vi "V1.0_UI.vi"() -> ()   [LabVIEW 2018]
uses:
  lib/Olympus IX BX Series/Olympus IX BX Series.lvlib
  <vilib>/MakerHub/LINX/LMH-LINX.lvlib
  lib/ARDUINO/VIs/Arduino.lvlib
  lib/SOLA/LabVIEW 2015 Library (32bit)/LumencorDLL32/LumencorDLL32.lvlib
  lib/TANGO Stage/TangoOWN.lvlib
  <userlib>/Tango_DLL/Tango_DLL.lvlib
  lib/ANDOR/Andor SDK/AndorSDK.lvlib
  lib/ANDOR/OwnVIs/AndorOWN.lvlib
  <vilib>/vision/NI_Vision_Development_Module.lvlib
  <vilib>/MakerHub/LINX/Public/Utilities/Open Serial.vi
  <vilib>/Utility/inputDevices.llb/closeKeyboard.vi
  <vilib>/Utility/inputDevices.llb/keyboardAcquire.vi
panel:
  in  "Filter":u16(ring) items=["UV ", "CFP", "GFP", "YFP", "RFP", "BF (empty)"]
  in  "Exposure":sgl=50.0 format="%#_g ms"
  out "exposure out":sgl
  out "accumulate out":sgl
  out "kinetic out":sgl
  out "Camera Temperature":sgl format="%.2f °C"
  in  "Single/\nMultiring?":bool
  in  "Image Name":string="TestIMG"
  out "Acq. Error Array":cluster{i32, string}[](array[cluster])
  in  "Live Mode":bool
  in  "Single Image":bool
  in  "Calibrate at Startup":bool
  out "keys pressed":T1(array[ring])
  out "Position List":i32[](listbox)
  in  "Down":bool
  in  "Left":bool
  in  "Up":bool
  in  "Right":bool
  in  "Clear Last Pos":bool
  in  "Save Pos":bool
  out "Boolean":bool
  in  "TANGO COM Port":refnum<visa-resource-name>="COM4"
  in  "SOLA COM Port":u32=5 max=10 step=1
  in  "Valve Port (Arduino)":refnum<visa-resource-name>="COM7"
  in  "IX 81 Port (IX2 UCB)":refnum<visa-resource-name>="IX2-UCB"
  out "Tango Connection\n Error":i32
  out "Y Limits":dbl[](array[numeric]) caption="Y Limits [µm]" format="%#_12f"
  out "X Limits":dbl[](array[numeric]) caption="X Limits [µm]" format="%#_10f"
  in  "Step Width [µm]":dbl=100.0 min=0.0 format="%#_6f"
  out "Position":dbl[](array[numeric]) caption="Position [µm]" format="%#_12f"
  out "Current z-Position":dbl
  in  "Direction (1: Down)":enum16{"Up", "Down", "Abs"}(ring)=enum."Abs"
  in  "Step (0.0 um)":dbl format="%.1f"
  out "Upper Limit":dbl
  out "Lower Limit":dbl
  in  "Light Source":u16(ring) items=["BF - Lamp", "SOLA"]
  in  "Intensity [%]":dbl(slide) scale=0.0..100.0 scale format="%.1f"
  in  "Prism Position (1: Bi)":enum16{"Bi", "Side"}(ring)=enum."Side"
  in  "Objective":enum16{"x 4", "x 10", "x 20", "x 40", "x 100"}(ring)=enum."x 10"
  in  "Shutter":bool
  in  "Enable Lamp":bool
  in  "Lamp Type (0: Transmitted)":enum16{"Transmitted", "Reflected"}(ring)
  out "Info":string caption="String"
  out "Image":T2(plugin-control)
  out "error out":errorcluster
  in  "Flush\nReagent":u16
  in  "Flush":bool
  in  "Pump Cycles":dbl=20.0
  in  "Frequency":dbl=50.0 format="%#_3f"
  in  "Pump On":bool
  in  "Feed On":bool
  in  "Feed Cycles":i32=20
  in  "Feed\nReagent":u16=2
  in  "Ring":u16
  in  "All Rings":bool
  in  "stop":bool
  # "Stage"
  # "X"
  # "Y"
  # "min"
  # "min"
  # "max"
  # "max"
  # "S"
  # "M"
  # "Initialization"
  # "Microscope"
  # "Valve Functions"
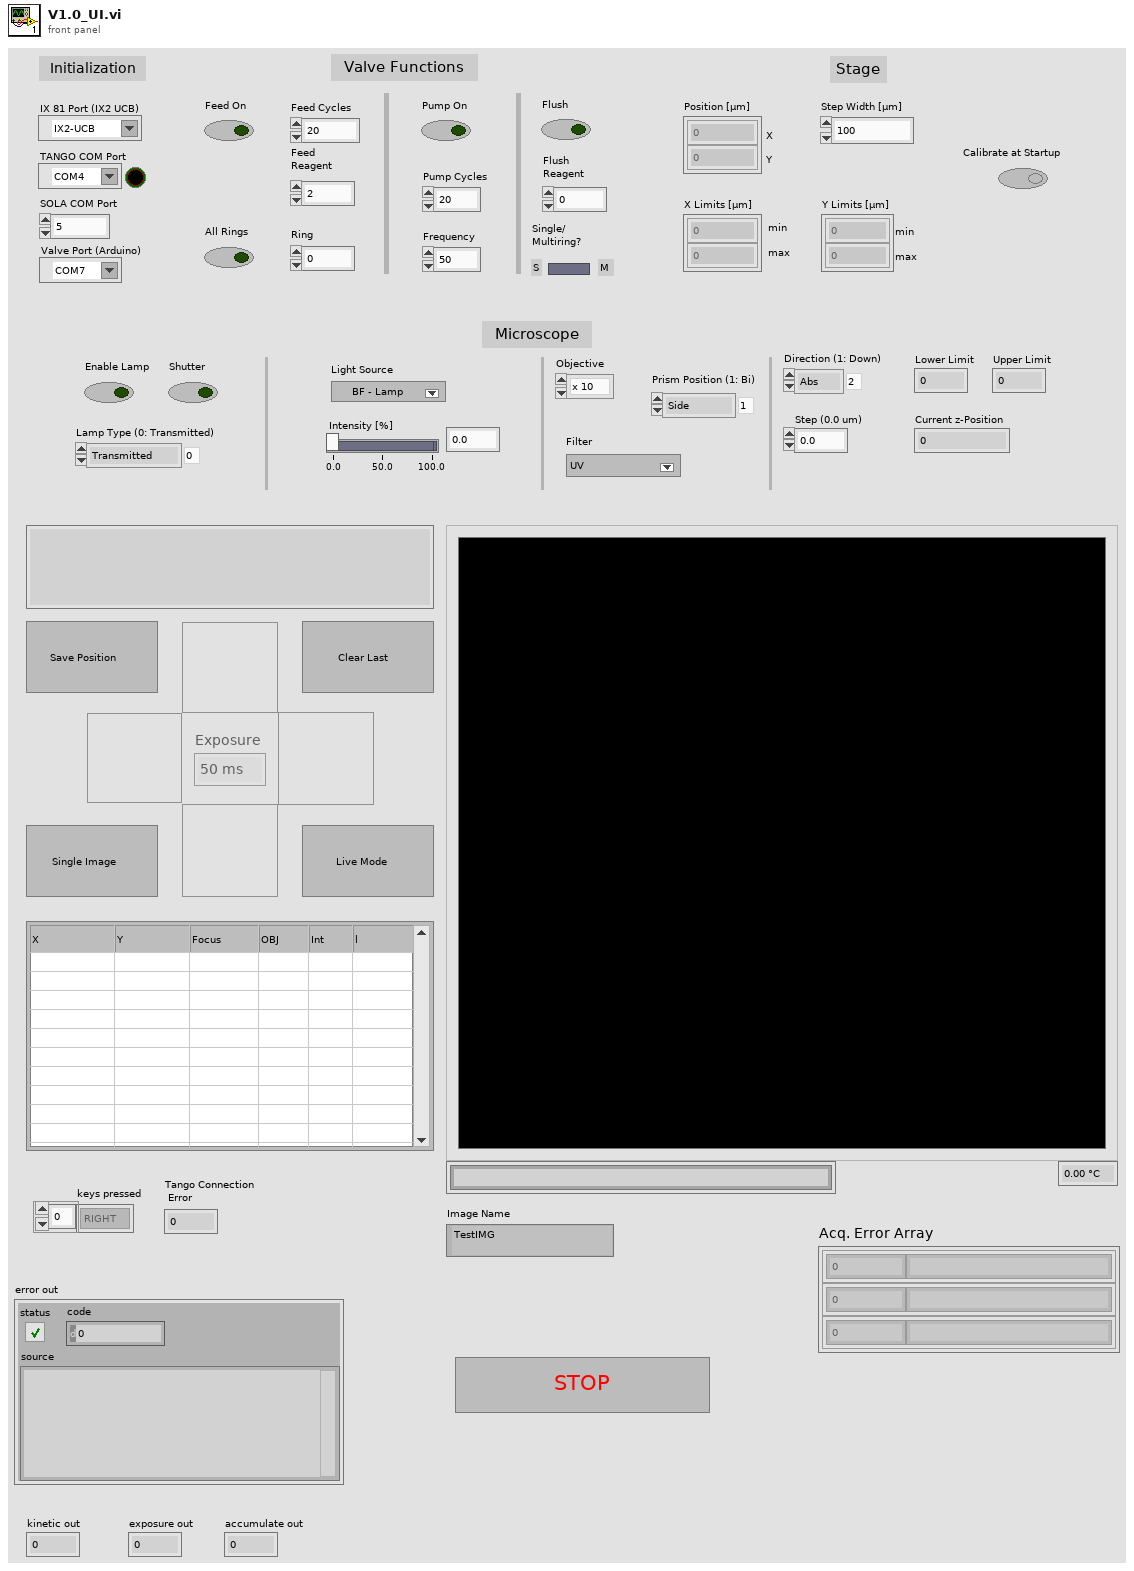
[diagram p1: front panel]
types:
  T1 = enum16{"0", "1", "2", "3", "4", "5", "6", "7", "8", "9", "A", "B", "C", "D", "E", "F", "G", "H", "I", "J", "K", "L", "M", "N", "O", "P", "Q", "R", "S", "T", "U", "V", "W", "X", "Y", "Z", "F1", "F2", "F3", "F4", "F5", "F6", "F7", "F8", "F9", "F10", "F11", "F12", "F13", "F14", "F15", "ADD", "BACK", "BACKSLASH", "CAPITAL", "COMMA", "DECIMAL", "DELETE", "DIVIDE", "DOWN", "END", "EQUALS", "ESCAPE", "GRAVE (`)", "HOME", "INSERT", "LBRACKET", "LCONTROL", "LEFT", "L ALT", "LSHIFT", "LWIN", "MINUS", "MULTIPLY", "NEXT", "NUMLOCK", "NUMPAD_0", "NUMPAD_1", "NUMPAD_2", "NUMPAD_3", "NUMPAD_4", "NUMPAD_5", "NUMPAD_6", "NUMPAD_7", "NUMPAD_8", "NUMPAD_9", "PAUSE", "PERIOD", "PRIOR (PG UP)", "RBRACKET", "RCONTROL", "RETURN", "RIGHT", "R ALT", "RSHIFT", "RWIN", "SCROLL", "SEMICOLON", "SLASH", "SPACE", "SUBTRACT", "TAB", "UP", "ENTER (num pad)", "' (quote)"}[]
  T2 = typedef "IMAQ Image.ctl" = refnum<image>
  T3 = enum32{"UV", "CFP", "GFP", "YFP", "RFP", "BF (empty)"}
  T4 = typedef "LMH-LINX.lvlib/LINX Ref.ctl" = cluster{"IO":T5, "Interface":T6, "LINX Device Config":T7}
  T5 = typedef "LMH-LINX.lvlib/Platform.ctl" = enum16{"Remote", "Local"}
  T6 = typedef "LMH-LINX.lvlib/Interface.ctl" = enum16{"Serial", "TCP"}
  T7 = typedef "LMH-LINX.lvlib/Device.lvlib/LINX Device Config.ctl" = cluster{"Interface":T6, "COM Port":refnum<visa-resource-name>, "TCP Configuration":T8, "Device Family":u8, "Device ID":u8, "Device Name":string, "TCP Ref":refnum<k5>, "Channels":T9}
  T8 = typedef "LMH-LINX.lvlib/Device.lvlib/TCP Config.ctl" = cluster{"IP Address":string, "Port":u16}
  T9 = typedef "LMH-LINX.lvlib/Channels.ctl" = cluster{"DI":u8[], "DO":u8[], "AI":u8[], "AO":u8[], "PWM":u8[], "QE":u8[], "UART":u8[], "I2C 2":u8[], "SPI":u8[], "CAN":u8[], "Servo":u8[], "AI Ref (V)":dbl, "AI Resolution (Bits)":u8, "AO Ref (V)":dbl, "AO Resolution (Bits)":u8}
  T10 = cluster{"X":dbl, "Y\nY":dbl, "Focus":dbl, "Objective":string, "filter":string, "Intensity":dbl}[]
  T11 = cluster{"pdX out":dbl, "pdY out":dbl, dbl, string, string, "Value":dbl}
  T12 = cluster{"pdX out":dbl, "pdY out":dbl, "Focus":dbl, "Objective":string, "filter":string, "Value":dbl}[]
  T13 = enum8{"Enabled", "Disabled", "Disabled and Grayed Out"}
  T14 = typedef "Image Type" = u32
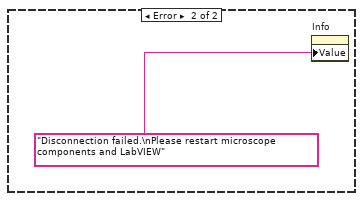
[diagram p2: hidden frame]
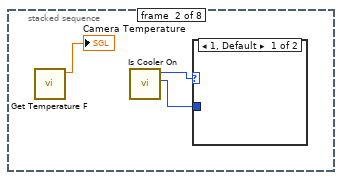
[diagram p3: hidden frame]
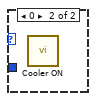
[diagram p4: hidden frame]
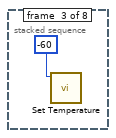
[diagram p5: hidden frame]
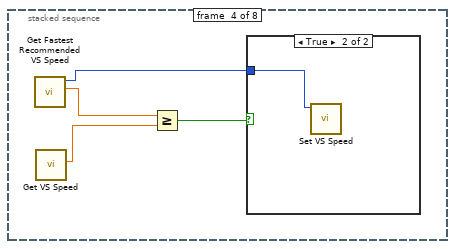
[diagram p6: hidden frame]
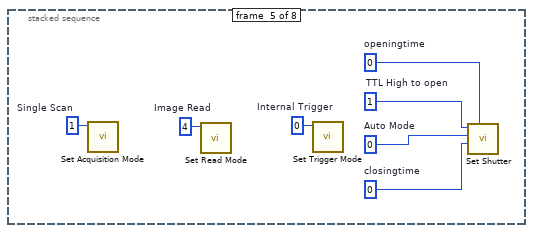
[diagram p8: hidden frame]
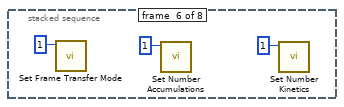
[diagram p9: hidden frame]
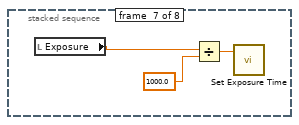
[diagram p10: hidden frame]
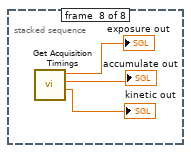
[diagram p11: hidden frame]
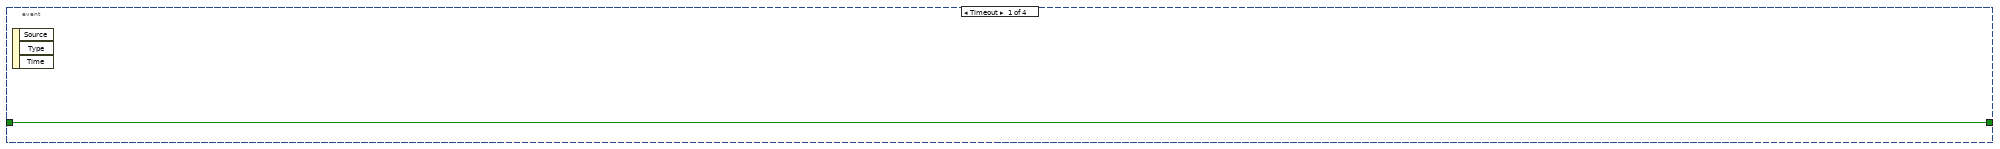
[diagram p12: hidden frame]
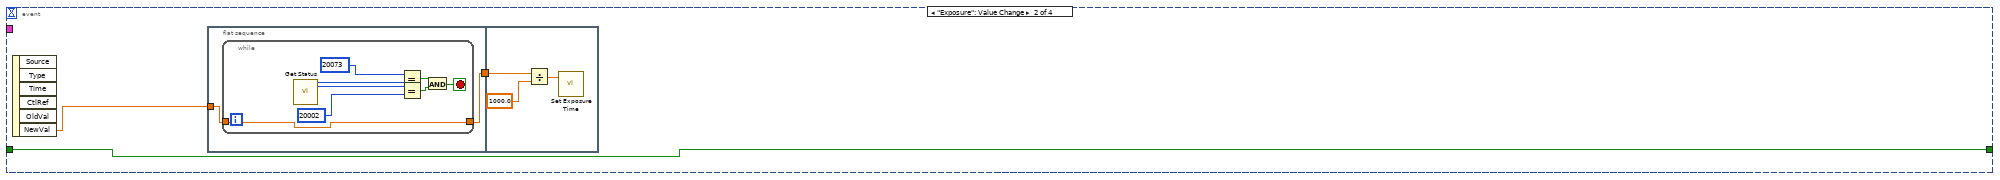
[diagram p13: hidden frame]
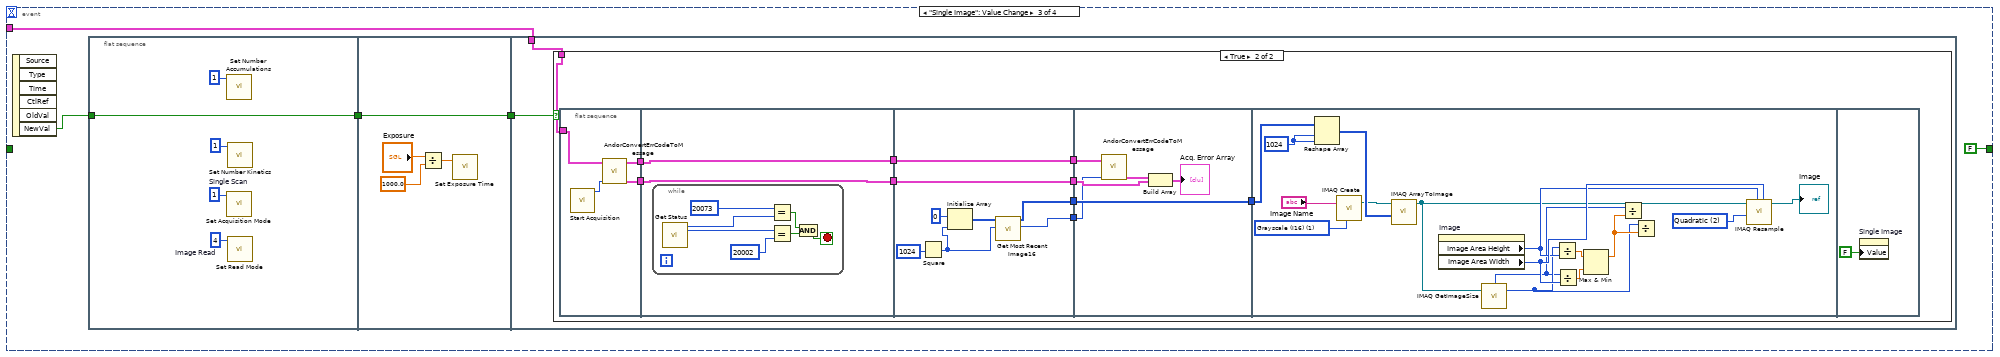
[diagram p14: hidden frame]
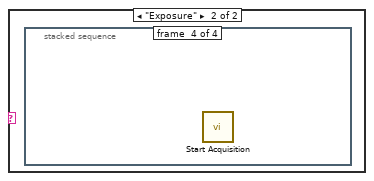
[diagram p17: hidden frame]
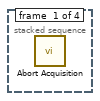
[diagram p18: hidden frame]
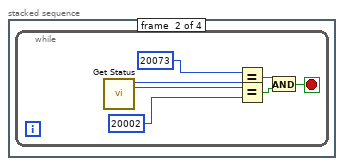
[diagram p19: hidden frame]
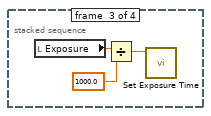
[diagram p20: hidden frame]
diagram:
  n1 = flat-sequence {
    tunnel: [w46] -> w22
    tunnel: [w47] -> w21
    tunnel: [w51] -> w20
    tunnel: [w43] -> w19
    tunnel: [w41] -> w18
    tunnel: w22 -> [w74]
    tunnel: [w74] -> w17
    tunnel: w21 -> [w73]
    tunnel: [w73] -> w15
    tunnel: w20 -> [w72]
    tunnel: [w72] -> w12
    tunnel: w19 -> [w71]
    tunnel: [w71] -> w10
    tunnel: w18 -> [w70]
    tunnel: [w70] -> w8
    tunnel: w17 -> [w81]
    tunnel: [w81] -> w16
    tunnel: w15 -> [w80]
    tunnel: [w80] -> w14
    tunnel: [w75] -> w13
    tunnel: w12 -> [w79]
    tunnel: [w79] -> w11
    tunnel: w10 -> [w78]
    tunnel: [w78] -> w9
    tunnel: w8 -> [w77]
    tunnel: w16 -> [w90]
    tunnel: [w104] -> w34
    tunnel: w14 -> [w172]
    tunnel: [w172] -> w32
    tunnel: w13 -> [w89]
    tunnel: [w96] -> w30
    tunnel: w11 -> [w171]
    tunnel: [w171] -> w28
    tunnel: w9 -> [w94]
    tunnel: [w94] -> w26
    tunnel: w34 -> [w195]
    tunnel: [w195] -> w33
    tunnel: w32 -> [w194]
    tunnel: [w194] -> w31
    tunnel: w30 -> [w189]
    tunnel: [w191] -> w29
    tunnel: w28 -> [w193]
    tunnel: [w193] -> w27
    tunnel: w26 -> [w192]
    tunnel: [w192] -> w25
    tunnel: [w187] -> w24
    tunnel: w33 -> [w209]
    tunnel: w31 -> [w207]
    tunnel: w29 -> [w208]
    tunnel: [w206] -> w39
    tunnel: [w205] -> w38
    tunnel: [w204] -> w37
    tunnel: w27 -> [w203]
    tunnel: [w202] -> w36
    tunnel: w25 -> [w200]
    tunnel: [w201] -> w35
    tunnel: w24 -> [w199]
    tunnel: [w198] -> w23
    tunnel: w39 -> [w785]
    tunnel: w38 -> [w779]
    tunnel: w37 -> [w771]
    tunnel: [w770] -> w4
    tunnel: w36 -> [w772]
    tunnel: w35 -> [w773]
    tunnel: w23 -> [w774]
    frame #0 {
      "Info" <- "Connecting..." ("Info")
    }
    frame #1 {
      w62 = 2  # Device Number (1: -Condensor      - Objective      - Lamp      - Shutter 2: - Z-Motion    - Autofocus)
      w61 = 1  # Device Number (1: -Condensor      - Objective      - Lamp      - Shutter 2: - Z-Motion    - Autofocus)
      n2 = call "Initialize.vi"("VISA Resource Name"="IX 81 Port (IX2 UCB)") -> ("VISA Resource Name Out"=w68:refnum<visa-resource-name>, "error out"=w67:errorcluster)  [unwired: 13 in]
      n3 = call "Login Device.vi"("error in (no error)"=w67, "Device Number (1)"=w61, "VISA Resource Name"=w68) -> ("error out"=w65:errorcluster, "VISA Resource Name Out"=w66:refnum<visa-resource-name>)  [unwired: 7 in]
      n4 = call "Login Device.vi"("error in (no error)"=w65, "Device Number (1)"=w62, "VISA Resource Name"=w66) -> ("error out"=w63:errorcluster, "VISA Resource Name Out"=w46:refnum<visa-resource-name>)  [unwired: 7 in]
      n5 = call-poly <vilib>:"Open.vi"("Error In"=w63, "Serial Port"="Valve Port (Arduino)") -> ("Error Out"=w60:errorcluster, "LINX Resource"=w47:T4)  [unwired: 7 in, 1 out]
      n6 = Decrement(x="SOLA COM Port") -> (x-1=w50:u32)
      n7 = call "lm Init.vi"("error in (no error)"=w60, "LETypeStr"="SOLA", "ComPort"=w50) -> ("error out"=w57:errorcluster, "function return"=w51:u32)  [unwired: 6 in, 1 out]
      n8 = call "lm Color Level.vi"("error in (no error)"=w57, "str_Level"="0", "str_Color"="WHITE") -> ("error out"=w53:errorcluster, "str_Color out"=w54:string)  [unwired: 6 in, 1 out]
      n9 = call "lm Color Enable.vi"("error in (no error)"=w53, "str_State"="OFF", "str_Color"=w54) -> ("error out"=w48:errorcluster)  [unwired: 6 in, 2 out]
      n10 = property on="Boolean" class="Bool (strict)"("Colors [4]"=cluster{u32, u32}[] [{16711680, 0}, {65280, 0}, {6710886, 0}, {6710886, 0}]) -> ()  [unwired: 2 in, 2 out]
      n11 = call "TangoConnectSub.vi"("error in (no error)"=w48, "VISA Refnum in"="TANGO COM Port") -> ("error out"=w41:errorcluster, "function return"=w45:i32, "plLSID out"=w43:i32)  [unwired: 7 in]
      "Tango Connection\n Error" <- w45
      n12 = Equal To 0?(x=w45) -> (x = 0?=→"Boolean":bool)
    }
    frame #2 {
    }
    frame #3 {
      n13 = property on="Info" class="Str"(error in=w77, "Value"="Connection to all devices successful." ("Info")) -> (error out=w75:errorcluster)  [unwired: 1 in, 1 out]
    }
    frame #4 {
      n14 = call "Set Active Objective.vi"("error in (no error)"=w89, "Objective Number (1)"=1, "Device Number (1)"=1, "VISA Resource Name"=w90) -> ("error out"=w92:errorcluster, "VISA Resource Name Out"=w91:refnum<visa-resource-name>)  [unwired: 6 in]
      n15 = case shown="True" "Calibrate at Startup" {
        tunnel: w94 -> [_ w180]
        tunnel: [w173 w179] -> w93
        tunnel: w92 -> [w173 w178]
        tunnel: [dbl[] [0.0, 80674.8] ("Y Limits") w177] -> w86
        tunnel: [dbl[] [0.0, 120822.0] ("X Limits") w176] -> w85
        frame False {
        }
        frame True {
          n16 = call "TangoCalibrate.vi"("error in (no error)"=w178, "plLSID in"=w180) -> ("error out"=w179:errorcluster, "X Limits"=w176:dbl[], "Y Limits"=w177:dbl[])  [unwired: 7 in]
        }
      }
      "X Limits" <- w85
      "Y Limits" <- w86
      n17 = call "OlympusQuery.vi"("error in (no error)"=w93, "Device Number\n(1: -Condensor\n     - Objective\n     - Lamp\n     - Shutter\n2: - Z-Motion\n   - Autofocus)"=1 ("Device Number\n(1: -Condensor\n     - Objective\n     - Lamp\n     - Shutter\n2: - Z-Motion\n   - Autofocus)"), "String"="SW OFF", "VISA Resource Name In"=w91) -> ("error out"=w101:errorcluster, "VISA Resource Name Out"=w102:refnum<visa-resource-name>)  [unwired: 5 in, 1 out]
      n18 = call "OlympusQuery.vi"("error in (no error)"=w101, "String"="LMPSW?", "VISA Resource Name In"=w102) -> ("error out"=w170:errorcluster, "Result"=w137:string, "VISA Resource Name Out"=w165:refnum<visa-resource-name>)  [unwired: 6 in]
      n19 = Equal?(x=w137, y="ON") -> (x = y?=w136:bool)
      n20 = property on="Enable Lamp" class="Bool (strict)"(error in=w170, "Value"=w136) -> (error out=w168:errorcluster)  [unwired: 1 in, 1 out]
      n21 = call "OlympusQuery.vi"("error in (no error)"=w168, "String"="LMP?", "VISA Resource Name In"=w165) -> ("error out"=w167:errorcluster, "Result"=w106:string, "VISA Resource Name Out"=w162:refnum<visa-resource-name>)  [unwired: 6 in]
      n22 = Decimal String To Number(string=w106, default (0L)=0.0 ("default (0 I32)")) -> (number=w108:dbl)  [unwired: 1 in, 1 out]
      n23 = Divide(x=w108, y=1.2 ("x")) -> (x/y=w134:dbl)
      n24 = property on="Intensity [%]" class="Slide (strict)"(error in=w167, "Value"=w134) -> (error out=w164:errorcluster)  [unwired: 1 in, 1 out]
      n25 = call "OlympusQuery.vi"("error in (no error)"=w164, "String"="SHUT1?", "VISA Resource Name In"=w162) -> ("error out"=w163:errorcluster, "Result"=w133:string, "VISA Resource Name Out"=w158:refnum<visa-resource-name>)  [unwired: 6 in]
      n26 = Equal?(x=w133, y="OUT") -> (x = y?=w131:bool)
      n27 = property on="Shutter" class="Bool (strict)"(error in=w163, "Value"=w131) -> (error out=w160:errorcluster)  [unwired: 1 in, 1 out]
      n28 = call "OlympusQuery.vi"("error in (no error)"=w160, "String"="LMPSEL?", "VISA Resource Name In"=w158) -> ("error out"=w159:errorcluster, "Result"=w130:string, "VISA Resource Name Out"=w155:refnum<visa-resource-name>)  [unwired: 6 in]
      n29 = Equal?(x=w130, y="DIA") -> (x = y?=w128:bool)
      n30 = Not(x=w128) -> (.not. x?=w127:bool)
      n31 = Boolean To (0,1)(Boolean=w127) -> (0, 1=w126:i16)
      n32 = property on="Lamp Type\n (0: Transmitted)" class="Enum (strict)"(error in=w159, "Value"=w126) -> (error out=w156:errorcluster)  [unwired: 1 in, 1 out]
      n33 = call "OlympusQuery.vi"("error in (no error)"=w156, "String"="MU?", "VISA Resource Name In"=w155) -> ("error out"=w82:errorcluster, "Result"=w125:string, "VISA Resource Name Out"=w98:refnum<visa-resource-name>)  [unwired: 6 in]
      n34 = Decimal String To Number(string=w125) -> (number=w124:i32)  [unwired: 2 in, 1 out]
      n35 = Decrement(x=w124) -> (x-1=w83:i32)
      n36 = local write "Filter"(w83) -> ()
      n37 = case shown="0, Default" w83 {
        tunnel: w82 -> [w182 w185]
        tunnel: [w181 w184] -> w97
        frame 0, Default {
          w183 = u16 1 items=["BF - Lamp", "SOLA"] ("Light Source")
          n38 = property on="Light Source" class="Ring (strict)"(error in=w182, "Value"=w183) -> (error out=w181:errorcluster)  [unwired: 1 in, 1 out]
        }
        frame 5 {
          w186 = u16 0 items=["BF - Lamp", "SOLA"] ("Light Source")
          n39 = property on="Light Source" class="Ring (strict)"(error in=w185, "Value"=w186) -> (error out=w184:errorcluster)  [unwired: 1 in, 1 out]
        }
      }
      n40 = call "OlympusQuery.vi"("error in (no error)"=w97, "String"="OB?", "VISA Resource Name In"=w98) -> ("error out"=w153:errorcluster, "Result"=w123:string, "VISA Resource Name Out"=w148:refnum<visa-resource-name>)  [unwired: 6 in]
      n41 = Decimal String To Number(string=w123) -> (number=w122:i32)  [unwired: 2 in, 1 out]
      n42 = Decrement(x=w122) -> (x-1=w99:i32)
      n43 = property on="Objective" class="Enum (strict)"(error in=w153, "Value"=w99) -> (error out=w151:errorcluster)  [unwired: 1 in, 1 out]
      n44 = call "OlympusQuery.vi"("error in (no error)"=w151, "String"="PRISM?", "VISA Resource Name In"=w148) -> ("error out"=w150:errorcluster, "Result"=w121:string, "VISA Resource Name Out"=w146:refnum<visa-resource-name>)  [unwired: 6 in]
      n45 = Decimal String To Number(string=w121) -> (number=w120:i32)  [unwired: 2 in, 1 out]
      n46 = Decrement(x=w120) -> (x-1=w119:i32)
      n47 = property on="Prism Position\n (1: Bi)" class="Enum (strict)"(error in=w150, "Value"=w119) -> (error out=w147:errorcluster)  [unwired: 1 in, 1 out]
      n48 = call "OlympusQuery.vi"("error in (no error)"=w147, "Device Number\n(1: -Condensor\n     - Objective\n     - Lamp\n     - Shutter\n2: - Z-Motion\n   - Autofocus)"=2 ("Device Number\n(1: -Condensor\n     - Objective\n     - Lamp\n     - Shutter\n2: - Z-Motion\n   - Autofocus)"), "String"="FARLMT 10", "VISA Resource Name In"=w146) -> ("error out"=w143:errorcluster, "VISA Resource Name Out"=w144:refnum<visa-resource-name>)  [unwired: 5 in, 1 out]
      n49 = call "OlympusQuery.vi"("error in (no error)"=w143, "Device Number\n(1: -Condensor\n     - Objective\n     - Lamp\n     - Shutter\n2: - Z-Motion\n   - Autofocus)"=2 ("Device Number\n(1: -Condensor\n     - Objective\n     - Lamp\n     - Shutter\n2: - Z-Motion\n   - Autofocus)"), "String"="NEARLMT 3000000", "VISA Resource Name In"=w144) -> ("error out"=w140:errorcluster, "VISA Resource Name Out"=w141:refnum<visa-resource-name>)  [unwired: 5 in, 1 out]
      n50 = call "OlympusQuery.vi"("error in (no error)"=w140, "Device Number\n(1: -Condensor\n     - Objective\n     - Lamp\n     - Shutter\n2: - Z-Motion\n   - Autofocus)"=2 ("Device Number\n(1: -Condensor\n     - Objective\n     - Lamp\n     - Shutter\n2: - Z-Motion\n   - Autofocus)"), "String"="POS?", "VISA Resource Name In"=w141) -> ("error out"=w112:errorcluster, "Result"=w113:string, "VISA Resource Name Out"=w111:refnum<visa-resource-name>)  [unwired: 5 in]
      n51 = Decimal String To Number(string=w113, default (0L)=0.0 ("default (0 I32)")) -> (number=→"Current z-Position":dbl)  [unwired: 1 in, 1 out]
      n52 = call "Configure Jog.vi"("VISA Resource Name"=w111, "Device Number (1)"=2, "Enabled (False)"=TRUE, "error in (no error)"=w112) -> ("VISA Resource Name Out"=w104:refnum<visa-resource-name>, "error out"=w96:errorcluster)  [unwired: 10 in]
      "Lower Limit" <- 3000000.0 ("default (0 I32)")
      "Upper Limit" <- 10.0 ("Upper Limit")
    }
    frame #5 {
      n53 = call <vilib>:"Intialize Keyboard.vi"("error in (no error)"=w189) -> ("error out"=w188:errorcluster, "device ID"=w187:refnum<k1>)  [unwired: 9 in]
      n54 = property on="Info" class="Str"(error in=w188, "Value"="Initialization Finished") -> (error out=w191:errorcluster)  [unwired: 1 in, 1 out]
    }
    frame #6 {
      w196 = T10 []  # Saved Positions
      w197 = ""  # Current Button
      n55 = while {
        shift-right: [w210] -> w204
        shift-left: w208 -> [w246]
        shift-right: [w243] -> w206
        shift-left: w207 -> [w244]
        shift-right: [w245] -> w205
        shift-left: w209 -> [w247]
        tunnel: w203 -> [w242]
        tunnel: [w241] -> w202
        shift-right: [w235] -> w201
        shift-left: w200 -> [w234]
        shift-right: [w232] -> w198
        shift-left: w199 -> [w231]
        shift-right: [w223] -> _
        shift-left: w197 -> [w230]
        shift-right: [w211] -> _
        shift-left: w196 -> [w213]
        stop <- w248 stop-if-true
        n56 = flat-sequence {
          tunnel: w247 -> [w257]
          tunnel: w246 -> [w256]
          tunnel: [w255] -> w240
          tunnel: [w254] -> w239
          tunnel: w244 -> [w253]
          tunnel: [w253] -> w238
          tunnel: w242 -> [w252]
          tunnel: [w252] -> w237
          tunnel: w234 -> [w251]
          tunnel: [w251] -> w236
          tunnel: [w250] -> w233
          tunnel: w231 -> [w250]
          tunnel: w240 -> [w429]
          tunnel: [w429] -> w229
          tunnel: w239 -> [w426]
          tunnel: w238 -> [w428]
          tunnel: w237 -> [w430]
          tunnel: [w430] -> w228
          tunnel: w236 -> [w420]
          tunnel: [w428] -> w227
          tunnel: w233 -> [w427]
          tunnel: [w425] -> w232
          tunnel: w230 -> [w423]
          tunnel: [w422] -> w226
          tunnel: [w421] -> w225
          tunnel: [w420] -> w224
          tunnel: w229 -> [w545]
          tunnel: [w545] -> w222
          tunnel: w228 -> [w544]
          tunnel: [w544] -> w220
          tunnel: [w540] -> w218
          tunnel: w227 -> [w543]
          tunnel: [w543] -> w216
          tunnel: w226 -> [w542]
          tunnel: w225 -> [w541]
          tunnel: w224 -> [w540]
          tunnel: [w539] -> w223
          tunnel: [w537] -> w214
          tunnel: w222 -> [w626]
          tunnel: [w621] -> w221
          tunnel: w220 -> [w630]
          tunnel: [w630] -> w219
          tunnel: w218 -> [w625]
          tunnel: [w625] -> w217
          tunnel: w216 -> [w629]
          tunnel: [w629] -> w215
          tunnel: w214 -> [w627]
          tunnel: w213 -> [w628]
          tunnel: [w623] -> w211
          tunnel: [w622] -> w212
          tunnel: w221 -> [w708]
          tunnel: w219 -> [w705]
          tunnel: w217 -> [w704]
          tunnel: w215 -> [w710]
          tunnel: w212 -> [w707]
          tunnel: [w705] -> w241
          tunnel: [w709] -> w243
          tunnel: [w706] -> w210
          tunnel: [w708] -> w245
          tunnel: [w704] -> w235
          frame #0 {
            w258 = 2  # Device Number (1: -Condensor      - Objective      - Lamp      - Shutter 2: - Z-Motion    - Autofocus)
            w259 = 1  # Device Number (1: -Condensor      - Objective      - Lamp      - Shutter 2: - Z-Motion    - Autofocus)
            n57 = event shown="[8] \"Step (0.0 um)\": Value Change" {
              selector: _ -> [_ _ _ _ _ _ _ _ _]
              dyn-events: _ -> [_ _ _ _ _ _ _ _ _]
              timeout: 1 -> [_ _ _ _ _ _ _ _ _]
              tunnel: w257 -> [w264 w309 w329 w357 w362 w371 w375 w383 w414]
              tunnel: w259 -> [_ _ _ _ w360 w372 _ _ _]
              tunnel: w258 -> [_ _ _ _ _ _ _ _ w413]
              tunnel: [w263 w310 w323 w356 w364 w367 w377 w382 w411] -> w254
              tunnel: [w262 w309 w324 w357 w365 w368 w378 w385 w412] -> w255
              tunnel: w256 -> [w261 w311 w327 w356 w361 w370 w376 w384 w415]
              event "Enable Lamp": Value Change {
                n58 = event-data() -> ()  [unwired: 1 in, 6 out]
                n59 = case shown="True" "Enable Lamp" {
                  selector: "Enable Lamp" -> [w268 w301]
                  tunnel: w264 -> [w271 w305]
                  tunnel: w261 -> [w267 w296]
                  tunnel: [w270 w304] -> w263
                  tunnel: [w269 w303] -> w262
                  frame True {
                    n60 = case shown="1" "Light Source" {
                      tunnel: w271 -> [w283 w294]
                      tunnel: w267 -> [w273 w293]
                      tunnel: [w274 w284] -> w270
                      tunnel: [w283 w292] -> w269
                      tunnel: w268 -> [w272 w290]
                      frame 1 {
                        n61 = property on="Intensity [%]" class="Slide (strict)"() -> ("Value"=w276:dbl)  [unwired: 2 in, 2 out]
                        n62 = Boolean To (0,1)(Boolean=w272) -> (0, 1=w279:i16)
                        n63 = Number To Decimal String(number=w276) -> (decimal integer string=w275:string)  [unwired: 1 in]
                        n64 = Index Array(array=string[] ["OFF", "ON"], index=w279) -> (element=w281:string)
                        n65 = call "lm Color Enable.vi"("error in (no error)"=w273, "str_State"=w281, "str_Color"="WHITE") -> ("error out"=w278:errorcluster, "str_Color out"=w277:string)  [unwired: 6 in, 1 out]
                        n66 = call "lm Color Level.vi"("error in (no error)"=w278, "str_Level"=w275, "str_Color"=w277) -> ("error out"=w274:errorcluster)  [unwired: 6 in, 2 out]
                      }
                      frame 0, Default {
                        n67 = property on="Intensity [%]" class="Slide (strict)"() -> ("Value"=w287:dbl)  [unwired: 2 in, 2 out]
                        n68 = Multiply(x=0.12, y=w287) -> (x*y=w289:dbl)
                        n69 = local write "Filter"(T3."BF (empty)" ("Filter")) -> ()
                        n70 = call "Configure Lamp.vi"("VISA Resource Name"=w294, "Lamp Intensity (1.0 V)"=w289, "Device Number (1)"=1, "Lamp Enabled (True)"=w290, "Lamp Type (0: Transmitted)"="Lamp Type (0: Transmitted)", "error in (no error)"=w293) -> ("VISA Resource Name Out"=w292:refnum<visa-resource-name>, "error out"=w284:errorcluster)  [unwired: 8 in]
                      }
                    }
                  }
                  frame False {
                    n71 = property on="Lamp Type (0: Transmitted)" class="Enum (strict)"(error in=w296) -> (error out=w295:errorcluster, "Value"=w297:enum16{"Transmitted", "Reflected"})  [unwired: 1 in, 1 out]
                    n72 = property on="Intensity [%]" class="Slide (strict)"(error in=w295, "Val(Sgnl)"=u16 0 ("Intensity [%]")) -> (error out=w300:errorcluster)  [unwired: 1 in, 1 out]
                    n73 = call "Configure Lamp.vi"("VISA Resource Name"=w305, "Lamp Intensity (1.0 V)"=0.0, "Device Number (1)"=1, "Lamp Enabled (True)"=w301, "Lamp Type (0: Transmitted)"=w297, "error in (no error)"=w300) -> ("VISA Resource Name Out"=w303:refnum<visa-resource-name>, "error out"=w304:errorcluster)  [unwired: 8 in]
                  }
                }
              }
              event "Light Source": Value Change {
                n74 = event-data() -> ("OldVal"=w307:u16, "NewVal"=w306:u16)  [unwired: 1 in, 4 out]
                n75 = Not Equal?(x=w307, y=w306) -> (x != y?=w308:bool)
                n76 = case shown="True" w308 {
                  tunnel: w306 -> [_ w315]
                  tunnel: w311 -> [w312 w314]
                  tunnel: [w312 w313] -> w310
                  frame False {
                  }
                  frame True {
                    n77 = case shown="0, Default" w315 {
                      tunnel: w314 -> [w319 w322]
                      tunnel: [w316 w322] -> w313
                      frame 0, Default {
                        n78 = call "lm Color Level.vi"("error in (no error)"=w319, "str_Level"="0", "str_Color"="WHITE") -> ("error out"=w317:errorcluster)  [unwired: 6 in, 2 out]
                        n79 = property on="Filter" class="Ring (strict)"(error in=w317, "Val(Sgnl)"=T3."BF (empty)" ("Value (Signaling)")) -> (error out=w316:errorcluster)  [unwired: 1 in, 1 out]
                      }
                      frame 1 {
                      }
                    }
                  }
                }
              }
              event "Intensity [%]": Value Change {
                n80 = event-data() -> ("NewVal"=w325:dbl)  [unwired: 1 in, 5 out]
                n81 = property on="Light Source" class="Ring (strict)"(error in=w327) -> (error out=w326:errorcluster, "Value"=w330:u16)  [unwired: 1 in, 1 out]
                n82 = case shown="1" w330 {
                  tunnel: w329 -> [w344 w355]
                  tunnel: [w337 w354] -> w323
                  tunnel: [w344 w353] -> w324
                  tunnel: TRUE -> [_ w351]
                  tunnel: w326 -> [w335 w348]
                  tunnel: w325 -> [w332 w346]
                  frame 1 {
                    n83 = Number To Decimal String(number=w332) -> (decimal integer string=w339:string)  [unwired: 1 in]
                    n84 = Greater Than 0?(x=w332) -> (x > 0?=w331:bool)
                    n85 = property on="Enable Lamp" class="Bool (strict)"() -> ("Value"=w341:bool)  [unwired: 2 in, 2 out]
                    n86 = And(x=w331, y=w341) -> (x .and. y?=w333:bool)
                    n87 = call "lm Color Level.vi"("error in (no error)"=w335, "str_Level"=w339, "str_Color"="WHITE") -> ("error out"=w338:errorcluster, "str_Color out"=w334:string)  [unwired: 6 in, 1 out]
                    n88 = Boolean To (0,1)(Boolean=w333) -> (0, 1=w340:i16)
                    n89 = Index Array(array=string[] ["OFF", "ON"], index=w340) -> (element=w342:string)
                    n90 = call "lm Color Enable.vi"("error in (no error)"=w338, "str_State"=w342, "str_Color"=w334) -> ("error out"=w337:errorcluster)  [unwired: 6 in, 2 out]
                  }
                  frame 0, Default {
                    n91 = property on="Lamp Type (0: Transmitted)" class="Enum (strict)"(error in=w348) -> (error out=w347:errorcluster, "Value"=w349:enum16{"Transmitted", "Reflected"})  [unwired: 1 in, 1 out]
                    n92 = Multiply(x=w346, y=0.12 ("x")) -> (x*y=w350:dbl)
                    n93 = call "Configure Lamp.vi"("VISA Resource Name"=w355, "Lamp Intensity (1.0 V)"=w350, "Device Number (1)"=1, "Lamp Enabled (True)"=w351, "Lamp Type (0: Transmitted)"=w349, "error in (no error)"=w347) -> ("VISA Resource Name Out"=w353:refnum<visa-resource-name>, "error out"=w354:errorcluster)  [unwired: 8 in]
                  }
                }
              }
              event Timeout {
                n94 = event-data() -> ()  [unwired: 1 in, 3 out]
              }
              event "Objective": Value Change {
                n95 = event-data() -> ()  [unwired: 1 in, 6 out]
                n96 = To Unsigned Long Integer(number="Objective") -> (unsigned 32bit integer=w358:u32)
                n97 = Increment(x=w358) -> (x+1=w359:u32)
                n98 = call "Set Active Objective.vi"("error in (no error)"=w361, "Objective Number (1)"=w359, "Device Number (1)"=w360, "VISA Resource Name"=w362) -> ("error out"=w364:errorcluster, "VISA Resource Name Out"=w365:refnum<visa-resource-name>)  [unwired: 6 in]
              }
              event "Shutter": Value Change {
                n99 = event-data() -> ()  [unwired: 1 in, 6 out]
                n100 = Boolean To (0,1)(Boolean="Shutter") -> (0, 1=w369:i16)
                n101 = call "Set Shutter Status Extended.vi"("VISA Resource Name"=w371, "Device Number (1)"=w372, "Shutter Status (0: Open)"=w369, "error in (no error)"=w370) -> ("VISA Resource Name Out"=w368:refnum<visa-resource-name>, "error out"=w367:errorcluster)  [unwired: 10 in]
              }
              event "Prism Position (1: Bi)": Value Change {
                n102 = event-data() -> ()  [unwired: 1 in, 6 out]
                n103 = To Unsigned Long Integer(number="Prism Position (1: Bi)") -> (unsigned 32bit integer=w373:u32)
                n104 = call "Select Prism.vi"("error in (no error)"=w376, "Prism Position (0: Bi)"=w373, "VISA Resource Name"=w375) -> ("error out"=w377:errorcluster, "VISA Resource Name Out"=w378:refnum<visa-resource-name>)  [unwired: 7 in]
              }
              event "Filter": Value Change {
                n105 = event-data() -> ("OldVal"=w380:u16, "NewVal"=w379:u16)  [unwired: 1 in, 4 out]
                n106 = Not Equal?(x=w380, y=w379) -> (x != y?=w381:bool)
                n107 = case shown="True" w381 {
                  tunnel: [w386 w389] -> w385
                  tunnel: w384 -> [w387 w396]
                  tunnel: w383 -> [w386 w395]
                  tunnel: [w387 w393] -> w382
                  frame False {
                  }
                  frame True {
                    n108 = local read "Filter"() -> (w388:u16)
                    n109 = To Unsigned Long Integer(number=w388) -> (unsigned 32bit integer=w391:u32)
                    n110 = Increment(x=w391) -> (x+1=w392:u32)
                    n111 = call "Select Filter Wheel.vi"("error in (no error)"=w396, "Filter Wheel Position (1)"=w392, "VISA Resource Name"=w395) -> ("error out"=w394:errorcluster, "VISA Resource Name Out"=w390:refnum<visa-resource-name>)  [unwired: 7 in]
                    n112 = case shown="5" w388 {
                      tunnel: w394 -> [w400 w407]
                      tunnel: [w402 w410] -> w393
                      tunnel: w390 -> [w399 w404]
                      tunnel: [w397 w404] -> w389
                      frame 0, Default {
                        w403 = u16 1 items=["BF - Lamp", "SOLA"] ("Light Source")
                        n113 = call "Set Lamp intensity.vi"("error in (no error)"=w400, "Lamp Intensity (1.0 V)"=0.0, "VISA Resource Name"=w399) -> ("error out"=w401:errorcluster, "VISA Resource Name Out"=w397:refnum<visa-resource-name>)  [unwired: 7 in]
                        n114 = property on="Light Source" class="Ring (strict)"(error in=w401, "Val(Sgnl)"=w403) -> (error out=w402:errorcluster)  [unwired: 1 in, 1 out]
                      }
                      frame 5 {
                        w409 = u16 0 items=["BF - Lamp", "SOLA"] ("Light Source")
                        n115 = call "lm Color Level.vi"("error in (no error)"=w407, "str_Level"="0", "str_Color"="WHITE") -> ("error out"=w408:errorcluster)  [unwired: 6 in, 2 out]
                        n116 = property on="Light Source" class="Ring (strict)"(error in=w408, "Val(Sgnl)"=w409) -> (error out=w410:errorcluster)  [unwired: 1 in, 1 out]
                      }
                    }
                  }
                }
              }
              event "Step (0.0 um)": Value Change {
                n117 = event-data() -> ()  [unwired: 1 in, 6 out]
                n118 = call "Move Focusing Unit.vi"("VISA Resource Name"=w414, "Device Number (1)"=w413, "Direction (1: Down)"="Direction (1: Down)", "Step (0.0 um)"="Step (0.0 um)", "error in (no error)"=w415) -> ("VISA Resource Name Out"=w412:refnum<visa-resource-name>, "error out"=w411:errorcluster)  [unwired: 9 in]
              }
            }
          }
          frame #1 {
            n119 = call-poly <vilib>:"Acquire Input Data.vi"("device ID"=w427, "error in (no error)"=w426) -> ("device ID"=w425:refnum<k1>, "keys pressed"=→"keys pressed":T1, "error out"=w418:errorcluster)  [unwired: 15 in]
            n120 = event shown="[2] \"Down\": Value Change" {
              selector: _ -> [_ _ _ _ _]
              dyn-events: _ -> [_ _ _ _ _]
              timeout: 1 -> [_ _ _ _ _]
              tunnel: [w433 w457 w482 w506 w536] -> w421
              tunnel: w420 -> [w435 w459 w484 w508 _]
              tunnel: w418 -> [w434 w458 w483 w507 w536]
              tunnel: w423 -> [_ _ w480 _ w535]
              tunnel: [w431 w455 w479 w504 w535] -> w422
              tunnel: w418 -> [_ _ _ _ _]
              event "Right": Value Change {
                n121 = event-data() -> ("NewVal"=w432:bool)  [unwired: 1 in, 5 out]
                n122 = case shown="True" w432 {
                  tunnel: w435 -> [_ w454]
                  tunnel: w434 -> [w437 w453]
                  tunnel: [w437 w452] -> w433
                  tunnel: ["" "Right"] -> w431
                  frame False {
                  }
                  frame True {
                    n123 = Multiply(x=-1.0, y="Step Width [µm]") -> (x*y=w440:dbl)
                    n124 = call <userlib>:"LSX Move Rel.vi"("bWait"=0, "dA"=0.0, "dZ"=0.0, "error in (no error)"=w453, "dY"=0.0, "dX"=w440, "lLSID"=w454) -> ("error out"=w442:errorcluster)  [unwired: 3 in, 1 out]
                    n125 = call <userlib>:"LSX Get Pos.vi"("lLSID"=w454, "error in (no error)"=w442) -> ("pdA out"=w443:dbl, "pdX out"=w446:dbl, "pdY out"=w445:dbl, "pdZ out"=w444:dbl, "error out"=w452:errorcluster)  [unwired: 8 in, 1 out]
                    n126 = Build Array(w446, w445, w444, w443) -> (→"Position":dbl[])
                  }
                }
              }
              event "Up": Value Change {
                n127 = event-data() -> ("NewVal"=w456:bool)  [unwired: 1 in, 5 out]
                n128 = case shown="True" w456 {
                  tunnel: w459 -> [_ w478]
                  tunnel: w458 -> [w461 w477]
                  tunnel: [w461 w476] -> w457
                  tunnel: ["" "Up"] -> w455
                  frame False {
                  }
                  frame True {
                    n129 = property on="Step Width [µm]" class="DigNum (strict)"() -> ("Value"=w464:dbl)  [unwired: 2 in, 2 out]
                    n130 = Multiply(x=-1.0, y=w464) -> (x*y=w466:dbl)
                    n131 = call <userlib>:"LSX Move Rel.vi"("bWait"=0, "dA"=0.0, "dZ"=0.0, "error in (no error)"=w477, "dY"=w466, "dX"=0.0 ("dY"), "lLSID"=w478) -> ("error out"=w468:errorcluster)  [unwired: 3 in, 1 out]
                    n132 = call <userlib>:"LSX Get Pos.vi"("lLSID"=w478, "error in (no error)"=w468) -> ("pdA out"=w469:dbl, "pdX out"=w472:dbl, "pdY out"=w471:dbl, "pdZ out"=w470:dbl, "error out"=w476:errorcluster)  [unwired: 8 in, 1 out]
                    n133 = Build Array(w472, w471, w470, w469) -> (w463:dbl[])
                    n134 = property on="Position" class="Arr (strict)"("Value"=w463) -> ()  [unwired: 2 in, 2 out]
                  }
                }
              }
              event "Down": Value Change {
                n135 = event-data() -> ("NewVal"=w481:bool)  [unwired: 1 in, 5 out]
                n136 = case shown="True" w481 {
                  tunnel: w484 -> [_ w503]
                  tunnel: w483 -> [w486 w502]
                  tunnel: [w486 w501] -> w482
                  tunnel: w480 -> [_ _]
                  tunnel: ["" "Down"] -> w479
                  frame False {
                  }
                  frame True {
                    n137 = property on="Step Width [µm]" class="DigNum (strict)"() -> ("Value"=w489:dbl)  [unwired: 2 in, 2 out]
                    n138 = Multiply(x=1.0, y=w489) -> (x*y=w491:dbl)
                    n139 = call <userlib>:"LSX Move Rel.vi"("bWait"=0, "dA"=0.0, "dZ"=0.0, "error in (no error)"=w502, "dY"=w491, "dX"=0.0 ("dY"), "lLSID"=w503) -> ("error out"=w493:errorcluster)  [unwired: 3 in, 1 out]
                    n140 = call <userlib>:"LSX Get Pos.vi"("lLSID"=w503, "error in (no error)"=w493) -> ("pdA out"=w494:dbl, "pdX out"=w497:dbl, "pdY out"=w496:dbl, "pdZ out"=w495:dbl, "error out"=w501:errorcluster)  [unwired: 8 in, 1 out]
                    n141 = Build Array(w497, w496, w495, w494) -> (w488:dbl[])
                    n142 = property on="Position" class="Arr (strict)"("Value"=w488) -> ()  [unwired: 2 in, 2 out]
                  }
                }
              }
              event "Left": Value Change {
                n143 = event-data() -> ("NewVal"=w505:bool)  [unwired: 1 in, 5 out]
                n144 = case shown="True" w505 {
                  tunnel: w508 -> [w510 w534]
                  tunnel: w507 -> [w512 w533]
                  tunnel: [w511 w532] -> w506
                  tunnel: ["" "Left"] -> w504
                  frame False {
                    n145 = call <userlib>:"LSX Get Pos.vi"("lLSID"=w510, "error in (no error)"=w512) -> ("pdA out"=w514:dbl, "pdX out"=w517:dbl, "pdY out"=w516:dbl, "pdZ out"=w515:dbl, "error out"=w511:errorcluster)  [unwired: 8 in, 1 out]
                    n146 = Build Array(w517, w516, w515, w514) -> (w513:dbl[])
                    n147 = property on="Position" class="Arr (strict)"("Value"=w513) -> ()  [unwired: 2 in, 2 out]
                  }
                  frame True {
                    n148 = property on="Step Width [µm]" class="DigNum (strict)"() -> ("Value"=w519:dbl)  [unwired: 2 in, 2 out]
                    n149 = Multiply(x=1.0, y=w519) -> (x*y=w522:dbl)
                    n150 = call <userlib>:"LSX Move Rel.vi"("bWait"=0, "dA"=0.0, "dZ"=0.0, "error in (no error)"=w533, "dY"=0.0, "dX"=w522, "lLSID"=w534) -> ("error out"=w523:errorcluster)  [unwired: 3 in, 1 out]
                    n151 = call <userlib>:"LSX Get Pos.vi"("lLSID"=w534, "error in (no error)"=w523) -> ("pdA out"=w524:dbl, "pdX out"=w527:dbl, "pdY out"=w526:dbl, "pdZ out"=w525:dbl, "error out"=w532:errorcluster)  [unwired: 8 in, 1 out]
                    n152 = Build Array(w527, w526, w525, w524) -> (w520:dbl[])
                    n153 = property on="Position" class="Arr (strict)"("Value"=w520) -> ()  [unwired: 2 in, 2 out]
                  }
                }
              }
              event Timeout {
                n154 = event-data() -> ()  [unwired: 1 in, 3 out]
              }
            }
          }
          frame #2 {
            n155 = event shown="[0] Timeout" {
              selector: _ -> [_]
              dyn-events: _ -> [_]
              timeout: 10 -> [_]
              tunnel: w542 -> [w550]
              tunnel: w541 -> [w549]
              tunnel: w540 -> [w548]
              tunnel: [w547] -> w539
              tunnel: [w546] -> w537
              event Timeout {
                n156 = event-data() -> ()  [unwired: 1 in, 3 out]
                n157 = case shown="\"\", Default" w550 {
                  selector: w550 -> [w551 w566 w583 w600 w617]
                  tunnel: w549 -> [w552 w568 w585 w602 w619]
                  tunnel: [w552 w569 w586 w603 w620] -> w546
                  tunnel: [w551 w566 w583 w600 w617] -> w547
                  tunnel: w548 -> [_ w567 w584 w601 w618]
                  frame "", Default {
                  }
                  frame "Up" {
                    n158 = property on="Step Width [µm]" class="DigNum (strict)"() -> ("Value"=w554:dbl)  [unwired: 2 in, 2 out]
                    n159 = Multiply(x=-1.0, y=w554) -> (x*y=w556:dbl)
                    n160 = call <userlib>:"LSX Move Rel.vi"("bWait"=0, "dA"=0.0, "dZ"=0.0, "error in (no error)"=w568, "dY"=w556, "dX"=0.0 ("dY"), "lLSID"=w567) -> ("error out"=w558:errorcluster)  [unwired: 3 in, 1 out]
                    n161 = call <userlib>:"LSX Get Pos.vi"("lLSID"=w567, "error in (no error)"=w558) -> ("pdA out"=w559:dbl, "pdX out"=w562:dbl, "pdY out"=w561:dbl, "pdZ out"=w560:dbl, "error out"=w569:errorcluster)  [unwired: 8 in, 1 out]
                    n162 = Build Array(w562, w561, w560, w559) -> (w553:dbl[])
                    n163 = property on="Position" class="Arr (strict)"("Value"=w553) -> ()  [unwired: 2 in, 2 out]
                  }
                  frame "Down" {
                    n164 = property on="Step Width [µm]" class="DigNum (strict)"() -> ("Value"=w571:dbl)  [unwired: 2 in, 2 out]
                    n165 = Multiply(x=1.0, y=w571) -> (x*y=w573:dbl)
                    n166 = call <userlib>:"LSX Move Rel.vi"("bWait"=0, "dA"=0.0, "dZ"=0.0, "error in (no error)"=w585, "dY"=w573, "dX"=0.0 ("dY"), "lLSID"=w584) -> ("error out"=w575:errorcluster)  [unwired: 3 in, 1 out]
                    n167 = call <userlib>:"LSX Get Pos.vi"("lLSID"=w584, "error in (no error)"=w575) -> ("pdA out"=w576:dbl, "pdX out"=w579:dbl, "pdY out"=w578:dbl, "pdZ out"=w577:dbl, "error out"=w586:errorcluster)  [unwired: 8 in, 1 out]
                    n168 = Build Array(w579, w578, w577, w576) -> (w570:dbl[])
                    n169 = property on="Position" class="Arr (strict)"("Value"=w570) -> ()  [unwired: 2 in, 2 out]
                  }
                  frame "Right" {
                    n170 = property on="Step Width [µm]" class="DigNum (strict)"() -> ("Value"=w590:dbl)  [unwired: 2 in, 2 out]
                    n171 = Multiply(x=-1.0, y=w590) -> (x*y=w588:dbl)
                    n172 = call <userlib>:"LSX Move Rel.vi"("bWait"=0, "dA"=0.0, "dZ"=0.0, "error in (no error)"=w602, "dY"=0.0, "dX"=w588, "lLSID"=w601) -> ("error out"=w592:errorcluster)  [unwired: 3 in, 1 out]
                    n173 = call <userlib>:"LSX Get Pos.vi"("lLSID"=w601, "error in (no error)"=w592) -> ("pdA out"=w593:dbl, "pdX out"=w596:dbl, "pdY out"=w595:dbl, "pdZ out"=w594:dbl, "error out"=w603:errorcluster)  [unwired: 8 in, 1 out]
                    n174 = Build Array(w596, w595, w594, w593) -> (w589:dbl[])
                    n175 = property on="Position" class="Arr (strict)"("Value"=w589) -> ()  [unwired: 2 in, 2 out]
                  }
                  frame "Left" {
                    n176 = property on="Step Width [µm]" class="DigNum (strict)"() -> ("Value"=w607:dbl)  [unwired: 2 in, 2 out]
                    n177 = Multiply(x=1.0, y=w607) -> (x*y=w605:dbl)
                    n178 = call <userlib>:"LSX Move Rel.vi"("bWait"=0, "dA"=0.0, "dZ"=0.0, "error in (no error)"=w619, "dY"=0.0, "dX"=w605, "lLSID"=w618) -> ("error out"=w609:errorcluster)  [unwired: 3 in, 1 out]
                    n179 = call <userlib>:"LSX Get Pos.vi"("lLSID"=w618, "error in (no error)"=w609) -> ("pdA out"=w610:dbl, "pdX out"=w613:dbl, "pdY out"=w612:dbl, "pdZ out"=w611:dbl, "error out"=w620:errorcluster)  [unwired: 8 in, 1 out]
                    n180 = Build Array(w613, w612, w611, w610) -> (w606:dbl[])
                    n181 = property on="Position" class="Arr (strict)"("Value"=w606) -> ()  [unwired: 2 in, 2 out]
                  }
                }
              }
            }
          }
          frame #3 {
            n182 = event shown="[0] Timeout" {
              selector: _ -> [_ _ _]
              dyn-events: _ -> [_ _ _]
              timeout: 1 -> [_ _ _]
              tunnel: w628 -> [w633 w642 w692]
              tunnel: w625 -> [_ w641 _]
              tunnel: w627 -> [w631 w640 w691]
              tunnel: w626 -> [w632 w639 w693]
              tunnel: [w633 w634 w686] -> w623
              tunnel: [w632 w638 w693] -> w621
              tunnel: [w631 w636 w687] -> w622
              event Timeout {
                n183 = event-data() -> ()  [unwired: 1 in, 3 out]
              }
              event "Save Pos": Value Change {
                n184 = event-data() -> ("NewVal"=w643:bool)  [unwired: 1 in, 5 out]
                n185 = case shown="True" w643 {
                  tunnel: w642 -> [w646 w658]
                  tunnel: w641 -> [_ w683]
                  tunnel: w640 -> [w644 w682]
                  tunnel: w639 -> [w645 w676]
                  tunnel: [w646 w656] -> w634
                  tunnel: [w645 w655] -> w638
                  tunnel: [w644 w654] -> w637
                  frame False {
                  }
                  frame True {
                    n186 = call <userlib>:"LSX Get Pos.vi"("lLSID"=w683, "error in (no error)"=w682) -> ("pdX out"=w684:dbl, "pdY out"=w685:dbl, "error out"=w677:errorcluster)  [unwired: 8 in, 3 out]
                    n187 = call "OlympusQuery.vi"("error in (no error)"=w677, "Device Number\n(1: -Condensor\n     - Objective\n     - Lamp\n     - Shutter\n2: - Z-Motion\n   - Autofocus)"=2 ("Device Number\n(1: -Condensor\n     - Objective\n     - Lamp\n     - Shutter\n2: - Z-Motion\n   - Autofocus)"), "String"="POS?", "VISA Resource Name In"=w676) -> ("error out"=w672:errorcluster, "Result"=w678:string, "VISA Resource Name Out"=w673:refnum<visa-resource-name>)  [unwired: 5 in]
                    n188 = Decimal String To Number(string=w678, default (0L)=0.0 ("default (0 I32)")) -> (number=w675:dbl)  [unwired: 1 in, 1 out]
                    n189 = call "OlympusQuery.vi"("error in (no error)"=w672, "Device Number\n(1: -Condensor\n     - Objective\n     - Lamp\n     - Shutter\n2: - Z-Motion\n   - Autofocus)"=1 ("Device Number\n(1: -Condensor\n     - Objective\n     - Lamp\n     - Shutter\n2: - Z-Motion\n   - Autofocus)"), "String"="OB?", "VISA Resource Name In"=w673) -> ("error out"=w668:errorcluster, "Result"=w674:string, "VISA Resource Name Out"=w660:refnum<visa-resource-name>)  [unwired: 5 in]
                    n190 = Decimal String To Number(string=w674) -> (number=w667:i32)  [unwired: 2 in, 1 out]
                    n191 = property on="Objective" class="Enum (strict)"(error in=w668) -> (error out=w659:errorcluster, "Strings []"=w669:string[])  [unwired: 1 in, 1 out]
                    n192 = Decrement(x=w667) -> (x-1=w666:i32)
                    n193 = Index Array(array=w669, index=w666) -> (element=w665:string)
                    n194 = call "OlympusQuery.vi"("error in (no error)"=w659, "Device Number\n(1: -Condensor\n     - Objective\n     - Lamp\n     - Shutter\n2: - Z-Motion\n   - Autofocus)"=1 ("Device Number\n(1: -Condensor\n     - Objective\n     - Lamp\n     - Shutter\n2: - Z-Motion\n   - Autofocus)"), "String"="MU?", "VISA Resource Name In"=w660) -> ("error out"=w648:errorcluster, "Result"=w664:string, "VISA Resource Name Out"=w655:refnum<visa-resource-name>)  [unwired: 5 in]
                    n195 = Decimal String To Number(string=w664) -> (number=w661:i32)  [unwired: 2 in, 1 out]
                    n196 = Decrement(x=w661) -> (x-1=w650:i32)
                    n197 = property on="Filter" class="Ring (strict)"(error in=w648) -> (error out=w647:errorcluster, "Strings []"=w649:string[])  [unwired: 1 in, 1 out]
                    n198 = Index Array(array=w649, index=w650) -> (element=w652:string)
                    n199 = property on="Intensity [%]" class="Slide (strict)"() -> ("Value"=w651:dbl)  [unwired: 2 in, 2 out]
                    n200 = Bundle("pdX out"=w684, "pdY out"=w685, w675, w665, w652, "Value"=w651) -> (w657:T11)  [unwired: 1 in]
                    n201 = property on="Save Pos" class="Bool (strict)"(error in=w647, "Value"=FALSE ("Save Pos")) -> (error out=w654:errorcluster)  [unwired: 1 in, 1 out]
                    n202 = Build Array (concatenate)(w658, w657) -> (w656:T12)
                  }
                }
                n203 = call "TangoPositions2MultiList.vi"("error in (no error)"=w637, "Saved Positions"=w634) -> ("error out"=w636:errorcluster, "Array"=w635:string[][])  [unwired: 8 in]
                n204 = property on="Position List" class="MCListbox (strict)"("ItemNames"=w635) -> ()  [unwired: 2 in, 2 out]
              }
              event "Clear Last Pos": Value Change {
                n205 = event-data() -> ("NewVal"=w690:bool)  [unwired: 1 in, 5 out]
                n206 = case shown="True" w690 {
                  tunnel: [w695 w701] -> w688
                  tunnel: w692 -> [w694 w700]
                  tunnel: [w694 w697] -> w686
                  tunnel: w691 -> [w695 w696]
                  frame False {
                  }
                  frame True {
                    n207 = Array Size(array=w700) -> (size(s)=w699:i32)
                    n208 = Decrement(x=w699) -> (x-1=w698:i32)
                    n209 = Delete From Array(array=w700, index=w698) -> (array with subset deleted=w697:T10)  [unwired: 1 in, 1 out]
                    n210 = property on="Clear Last Pos" class="Bool (strict)"(error in=w696, "Value"=FALSE ("Clear Last Pos")) -> (error out=w701:errorcluster)  [unwired: 1 in, 1 out]
                  }
                }
                n211 = call "TangoPositions2MultiList.vi"("error in (no error)"=w688, "Saved Positions"=w686) -> ("error out"=w687:errorcluster, "Array"=w689:string[][])  [unwired: 8 in]
                n212 = property on="Position List" class="MCListbox (strict)"("ItemNames"=w689) -> ()  [unwired: 2 in, 2 out]
              }
            }
          }
          frame #4 {
            n213 = event shown="[0] \"Feed On\": Value Change" {
              selector: _ -> [_ _ _ _ _ _]
              dyn-events: _ -> [_ _ _ _ _ _]
              timeout: 1 -> [_ _ _ _ _ _]
              tunnel: w707 -> [w717 w731 w735 w738 w744 w761]
              tunnel: w710 -> [w716 w732 _ _ w743 w760]
              tunnel: [w714 w731 w734 w737 w741 w758] -> w706
              tunnel: [w713 w732 _ _ w742 w759] -> w709
              tunnel: "Single/\nMultiring?" -> [w712 _ _ _ w739 w756]
              event "Feed On": Value Change {
                n214 = event-data() -> ()  [unwired: 1 in, 6 out]
                n215 = case shown="True" "Feed On" {
                  tunnel: w717 -> [w718 w722]
                  tunnel: w716 -> [w719 w730]
                  tunnel: [w718 w728] -> w714
                  tunnel: [w719 w723] -> w713
                  tunnel: w712 -> [_ w720]
                  frame False {
                  }
                  frame True {
                    n216 = call "ArdnoFeed.vi"("LINX Resource"=w730, "Single / Multiring?"=w720, "Channel"="Feed\nReagent", "Ring"="Ring", "Feed Cycles"="Feed Cycles", "error in (no error)"=w722, "All Rings"="All Rings") -> ("LINX Resource out"=w723:T4, "error out"=w729:errorcluster)  [unwired: 7 in]
                    n217 = property on="Feed On" class="Bool (strict)"(error in=w729, "Value"=FALSE) -> (error out=w728:errorcluster)  [unwired: 1 in, 1 out]
                  }
                }
              }
              event Timeout {
                n218 = event-data() -> ()  [unwired: 1 in, 3 out]
              }
              event "Flush\nReagent": Value Change {
                n219 = event-data() -> ("NewVal"=w733:u16)  [unwired: 1 in, 5 out]
                n220 = property on="Feed\nReagent" class="DigNum (strict)"(error in=w735, "Value"=w733) -> (error out=w734:errorcluster)  [unwired: 1 in, 1 out]
              }
              event "Feed\nReagent": Value Change {
                n221 = event-data() -> ("NewVal"=w736:u16)  [unwired: 1 in, 5 out]
                n222 = property on="Flush\nReagent" class="DigNum (strict)"(error in=w738, "Value"=w736) -> (error out=w737:errorcluster)  [unwired: 1 in, 1 out]
              }
              event "Pump On": Value Change {
                n223 = event-data() -> ()  [unwired: 1 in, 6 out]
                n224 = case shown="True" "Pump On" {
                  tunnel: w744 -> [w745 w750]
                  tunnel: w743 -> [w746 w753]
                  tunnel: [w745 w755] -> w741
                  tunnel: [w746 w748] -> w742
                  tunnel: w739 -> [_ w747]
                  frame False {
                  }
                  frame True {
                    n225 = call "ArdnoPump.vi"("LINX Resource"=w753, "Pump Cycles"="Pump Cycles", "Pump Frequency"="Frequency", "error in (no error)"=w750, "Single/\nMultiring?"=w747) -> ("LINX Resource out"=w748:T4, "error out"=w749:errorcluster)
                    n226 = property on="Pump On" class="Bool (strict)"(error in=w749, "Value"=FALSE) -> (error out=w755:errorcluster)  [unwired: 1 in, 1 out]
                  }
                }
              }
              event "Flush": Value Change {
                n227 = event-data() -> ()  [unwired: 1 in, 6 out]
                n228 = case shown="True" "Flush" {
                  tunnel: w761 -> [w762 w767]
                  tunnel: w760 -> [w763 w769]
                  tunnel: [w762 w766] -> w758
                  tunnel: [w763 w765] -> w759
                  tunnel: w756 -> [_ w764]
                  frame False {
                  }
                  frame True {
                    n229 = call "ArdnoFlush.vi"("error in (no error)"=w767, "Single / Multivalve?"=w764, "Channel"="Flush\nReagent", "LINX Resource"=w769) -> ("error out"=w766:errorcluster, "LINX Resource out"=w765:T4)  [unwired: 6 in]
                  }
                }
              }
            }
          }
        }
        n230 = Or(x=w210, y="stop") -> (x .or. y?=w248:bool)
      }
    }
    frame #7 {
      n231 = call "Logout Device.vi"("Device Number (1)"=1, "VISA Resource Name"=w779) -> ("error out"=w780:errorcluster, "VISA Resource Name Out"=w787:refnum<visa-resource-name>)  [unwired: 8 in]
      n232 = call "Logout Device.vi"("Device Number (1)"=2, "VISA Resource Name"=w787) -> ("error out"=w781:errorcluster, "VISA Resource Name Out"=w788:refnum<visa-resource-name>)  [unwired: 8 in]
      n233 = call <vilib>:"Close.vi"("VISA Resource Name"=w788) -> ("error out"=w782:errorcluster)  [unwired: 14 in]
      n234 = call <vilib>:"Close.vi"("LINX Resource"=w785) -> ("Error Out"=w783:errorcluster)  [unwired: 10 in]
      n235 = call "lm Shut Down.vi"("hSerial"=w772) -> ("error out"=w784:errorcluster)  [unwired: 9 in, 1 out]
      n236 = call <userlib>:"LSX Disconnect.vi"("lLSID"=w773) -> ("error out"=w777:errorcluster)  [unwired: 9 in, 1 out]
      n237 = call-poly <vilib>:"Close Input Device.vi"("device ID"=w774) -> ("error out"=w775:errorcluster)  [unwired: 1 in, 8 out]
      n238 = call <userlib>:"LSX Free LSID.vi"("error in (no error)"=w777, "lLSID"=w773) -> ("error out"=w776:errorcluster)  [unwired: 8 in, 1 out]
      n239 = Merge Errors(w775, w776, w784, w783, w782, w781, w780, w771) -> (w770:errorcluster)
    }
  }
  n240 = flat-sequence {
    tunnel: [w789] -> w7
    tunnel: w7 -> [w818]
    tunnel: [w816] -> w2
    tunnel: [w942] -> w5
    tunnel: w2 -> [w940]
    frame #0 {
      n241 = stacked-sequence {
        frame #0 {
          n242 = call "Initialize.vi"("dir"="C:\\Users\\e14user\\Documents\\LabVIEW software\\GitRepo\\lib\\ANDOR\\Libraries") -> ()  [unwired: 9 in, 2 out]
        }
        frame #1 {
          n243 = call "Get Temperature F.vi"() -> ("temperature out"=→"Camera Temperature":sgl)  [unwired: 10 in, 1 out]
          n244 = call "Is Cooler On.vi"() -> ("function return"=w791:u32, "iCoolerStatus out"=w792:i32)  [unwired: 10 in]
          n245 = case shown="1, Default" w792 {
            tunnel: w791 -> [_ _]
            frame 1, Default {
            }
            frame 0 {
              n246 = call "Cooler ON.vi"() -> ()  [unwired: 11 in, 1 out]
            }
          }
        }
        frame #2 {
          n247 = call "Set Temperature.vi"("temperature"=-60) -> ()  [unwired: 10 in, 1 out]
        }
        frame #3 {
          n248 = call "Get Fastest Recommended VS Speed.vi"() -> ("speed out"=w798:sgl, "index out"=w795:i32)  [unwired: 9 in, 1 out]
          n249 = call "Get VS Speed.vi"() -> ("speed out"=w797:sgl)  [unwired: 10 in, 1 out]
          n250 = Greater Or Equal?(x=w798, y=w797) -> (x >= y?=w796:bool)
          n251 = case shown="True" w796 {
            tunnel: w795 -> [_ w799]
            frame False {
            }
            frame True {
              n252 = call "Set VS Speed.vi"("index"=w799) -> ()  [unwired: 10 in, 1 out]
            }
          }
        }
        frame #4 {
          w805 = 0  # openingtime
          w803 = 0  # Auto Mode
          w804 = 1  # TTL High to open
          w806 = 0  # closingtime
          w802 = 0  # Internal Trigger
          w800 = 1  # Single Scan
          w801 = 4  # Image Read
          n253 = call "Set Acquisition Mode.vi"("mode"=w800) -> ()  [unwired: 10 in, 1 out]
          n254 = call "Set Read Mode.vi"("mode"=w801) -> ()  [unwired: 10 in, 1 out]
          n255 = call "Set Trigger Mode.vi"("mode"=w802) -> ()  [unwired: 10 in, 1 out]
          n256 = call "Set Shutter.vi"("openingtime"=w805, "closingtime"=w806, "mode"=w803, "typ"=w804) -> ()  [unwired: 7 in, 1 out]
        }
        frame #5 {
          n257 = call "Set Frame Transfer Mode.vi"("mode"=1) -> ()  [unwired: 10 in, 1 out]
          n258 = call "Set Number Accumulations.vi"("number"=1) -> ()  [unwired: 10 in, 1 out]
          n259 = call "Set Number Kinetics.vi"("number"=1) -> ()  [unwired: 10 in, 1 out]
        }
        frame #6 {
          n260 = local read "Exposure"() -> (w810:sgl)
          n261 = Divide(x=w810, y=sgl 1000.0) -> (x/y=w812:sgl)
          n262 = call "Set Exposure Time.vi"("time"=w812) -> ()  [unwired: 10 in, 1 out]
        }
        frame #7 {
          n263 = call "Get Acquisition Timings.vi"() -> ("kinetic out"=→"kinetic out":sgl, "accumulate out"=→"accumulate out":sgl, "exposure out"=→"exposure out":sgl)  [unwired: 8 in, 1 out]
        }
      }
      n264 = call "AndorCreaterErrorCluster.vi"() -> ("Array"=w789:cluster{i32, string}[])  [unwired: 11 in]
    }
    frame #1 {
      n265 = while {
        tunnel: 1 -> [w825]
        tunnel: w818 -> [w820]
        shift-right: [w822] -> _
        shift-left: FALSE -> [w823]
        tunnel: [w820] -> w816
        stop <- w826 stop-if-true
        n266 = event shown="[3] \"Live Mode\": Value Change" {
          selector: _ -> [_ _ _ _]
          dyn-events: _ -> [_ _ _ _]
          timeout: w825 -> [_ _ _ _]
          tunnel: w820 -> [_ _ w848 _]
          tunnel: [w828 w831 FALSE w915] -> w824
          tunnel: w823 -> [w828 w831 _ _]
          event Timeout {
            n267 = event-data() -> ()  [unwired: 1 in, 3 out]
          }
          event "Exposure": Value Change {
            n268 = event-data() -> ("NewVal"=w829:sgl)  [unwired: 1 in, 5 out]
            n269 = flat-sequence {
              tunnel: [w832] -> w830
              tunnel: w829 -> [w833]
              tunnel: w830 -> [w842]
              frame #0 {
                n270 = while {
                  tunnel: w833 -> [w834]
                  tunnel: [w834] -> w832
                  stop <- w835 stop-if-true
                  n271 = call "Get Status.vi"() -> ("function return"=w841:u32, "status out"=w838:i32)  [unwired: 10 in]
                  n272 = Equal?(x=20073 ("status out"), y=w838) -> (x = y?=w837:bool)
                  n273 = Equal?(x=w841, y=20002 ("x")) -> (x = y?=w836:bool)
                  n274 = And(x=w837, y=w836) -> (x .and. y?=w835:bool)
                }
              }
              frame #1 {
                n275 = Divide(x=w842, y=sgl 1000.0) -> (x/y=w844:sgl)
                n276 = call "Set Exposure Time.vi"("time"=w844) -> ()  [unwired: 10 in, 1 out]
              }
            }
          }
          event "Single Image": Value Change {
            n277 = event-data() -> ("NewVal"=w849:bool)  [unwired: 1 in, 5 out]
            n278 = flat-sequence {
              tunnel: w849 -> [w854]
              tunnel: [w854] -> w845
              tunnel: [w858] -> w846
              tunnel: w845 -> [w858]
              tunnel: w848 -> [w859]
              tunnel: w846 -> [w860]
              frame #0 {
                w852 = 1  # Single Scan
                w853 = 4  # Image Read
                n279 = call "Set Number Accumulations.vi"("number"=1) -> ()  [unwired: 10 in, 1 out]
                n280 = call "Set Acquisition Mode.vi"("mode"=w852) -> ()  [unwired: 10 in, 1 out]
                n281 = call "Set Number Kinetics.vi"("number"=1) -> ()  [unwired: 10 in, 1 out]
                n282 = call "Set Read Mode.vi"("mode"=w853) -> ()  [unwired: 10 in, 1 out]
              }
              frame #1 {
                n283 = Divide(x="Exposure", y=sgl 1000.0) -> (x/y=w857:sgl)
                n284 = call "Set Exposure Time.vi"("time"=w857) -> ()  [unwired: 10 in, 1 out]
              }
              frame #2 {
                n285 = case shown="True" w860 {
                  tunnel: w859 -> [_ w870]
                  frame False {
                  }
                  frame True {
                    n286 = flat-sequence {
                      tunnel: w870 -> [w871]
                      tunnel: [w873] -> w869
                      tunnel: [w872] -> w868
                      tunnel: w869 -> [w875]
                      tunnel: w868 -> [w876]
                      tunnel: [w876] -> w867
                      tunnel: [w875] -> w866
                      tunnel: w867 -> [w891]
                      tunnel: w866 -> [w890]
                      tunnel: [w891] -> w865
                      tunnel: [w890] -> w864
                      tunnel: [w888] -> w863
                      tunnel: [w887] -> w862
                      tunnel: w865 -> [w894]
                      tunnel: w864 -> [w892]
                      tunnel: w863 -> [w893]
                      tunnel: w862 -> [w897]
                      tunnel: [w897] -> w861
                      tunnel: w861 -> [w898]
                      frame #0 {
                        n287 = call "Start Acquisition.vi"() -> ("function return"=w874:u32)  [unwired: 11 in]
                        n288 = call "AndorConvertErrCodeToMessage.vi"("function return"=w874, "Array"=w871) -> ("Element Return"=w872:cluster{i32, string}, "Array out"=w873:cluster{i32, string}[])  [unwired: 8 in]
                      }
                      frame #1 {
                        n289 = while {
                          stop <- w877 stop-if-true
                          n290 = call "Get Status.vi"() -> ("function return"=w883:u32, "status out"=w880:i32)  [unwired: 10 in]
                          n291 = Equal?(x=20073 ("status out"), y=w880) -> (x = y?=w879:bool)
                          n292 = Equal?(x=w883, y=20002 ("x")) -> (x = y?=w878:bool)
                          n293 = And(x=w879, y=w878) -> (x .and. y?=w877:bool)
                        }
                      }
                      frame #2 {
                        n294 = Square(x=1024) -> (x^2=w886:i32)
                        n295 = Initialize Array(0 ("element"), w886) -> (w884:i32[])
                        n296 = call "Get Most Recent Image16.vi"("size"=w886, "arr"=w884) -> ("function return"=w888:u32, "arr out"=w887:u16[])  [unwired: 7 in, 1 out]
                      }
                      frame #3 {
                        n297 = call "AndorConvertErrCodeToMessage.vi"("function return"=w893, "Array"=w892) -> ("Element Return"=w895:cluster{i32, string})  [unwired: 8 in, 1 out]
                        n298 = Build Array(w895, w894) -> (→"Acq. Error Array":cluster{i32, string}[])
                      }
                      frame #4 {
                        w901 = u32 2 items=["Zero Order", "Bi-Linear", "Quadratic", "Cubic Spline"] ("Interpolation Type")
                        w900 = T14 1 items=["Grayscale (U8)", "Grayscale (I16)", "Grayscale (SGL)", "Complex (CSG)", "RGB (U32)", "HSL (U32)", "RGB (U64)", "Grayscale (U16)"] ("Image Type")
                        w899 = 1024 ("dimension size")
                        n299 = Reshape Array(w898, w899, w899) -> (w904:u16[][])
                        n300 = call "IMAQ Create"("Image Name"="Image Name", "Image Type"=w900) -> ("New Image"=w902:T2)  [unwired: 3 in, 1 out]
                        n301 = call "IMAQ ArrayToImage"("Image Pixels (I16)"=w904, "Image"=w902) -> ("Image Out"=w911:T2)  [unwired: 8 in, 1 out]
                        n302 = property on="Image" class="ImageControl"() -> ("Image Area Height"=w912:u32, "Image Area Width"=w913:u32)  [unwired: 2 in, 2 out]
                        n303 = call "IMAQ GetImageSize"("Image"=w911) -> ("Y Resolution"=w908:i32, "X Resolution"=w907:i32)  [unwired: 3 in, 1 out]
                        n304 = Divide(x=w908, y=w912) -> (x/y=w905:dbl)
                        n305 = Divide(x=w907, y=w913) -> (x/y=w906:dbl)
                        n306 = Max & Min(x=w905, y=w906) -> (max(x,y)=w909:dbl)  [unwired: 1 out]
                        n307 = Divide(x=w907, y=w909) -> ()  [unwired: 1 out]
                        n308 = Divide(x=w908, y=w909) -> ()  [unwired: 1 out]
                        n309 = call "IMAQ Resample"("X Resolution"=w913, "Y Resolution"=w912, "Interpolation Type"=w901, "Image Src"=w911) -> ("Image Dst Out"=→"Image":T2)  [unwired: 6 in, 1 out]
                      }
                      frame #5 {
                        n310 = property on="Single Image" class="Bool (strict)"("Value"=FALSE ("Single Image")) -> ()  [unwired: 2 in, 2 out]
                      }
                    }
                  }
                }
              }
            }
          }
          event "Live Mode": Value Change {
            n311 = event-data() -> ("NewVal"=w915:bool)  [unwired: 1 in, 5 out]
          }
        }
        n312 = case shown="True" w824 {
          selector: w824 -> [w916 _]
          tunnel: [w916 FALSE] -> w822
          frame False {
          }
          frame True {
            n313 = flat-sequence {
              frame #0 {
                n314 = property on="Exposure" class="DigNum (strict)"("DisabledEnum"=T13."Disabled and Grayed Out" ("Disabled")) -> ()  [unwired: 2 in, 2 out]
              }
              frame #1 {
                w919 = 4  # Image
                n315 = call "Set Read Mode.vi"("mode"=w919) -> ()  [unwired: 10 in, 1 out]
              }
              frame #2 {
                n316 = call "Set Kinetic Cycle Time.vi"("time"=sgl 0.0) -> ()  [unwired: 10 in, 1 out]
              }
              frame #3 {
                w921 = 5  # Run till abort
                n317 = call "Set Acquisition Mode.vi"("mode"=w921) -> ()  [unwired: 10 in, 1 out]
              }
              frame #4 {
                n318 = call "Start Acquisition.vi"() -> ()  [unwired: 11 in, 1 out]
              }
              frame #5 {
                n319 = while {
                  stop <- w923 stop-if-true
                  n320 = case shown="\"\", Default" "" {
                    frame "", Default {
                      n321 = local read "Image Name"() -> (w927:string)
                      n322 = call "AndorLiveMode.vi"("Image Name"=w927) -> ("Image"=w928:T2)  [unwired: 9 in, 1 out]
                      n323 = local write "Image"(w928) -> ()
                    }
                    frame "Exposure" {
                      n324 = stacked-sequence {
                        frame #0 {
                          n325 = call "Abort Acquisition.vi"() -> ()  [unwired: 11 in, 1 out]
                        }
                        frame #1 {
                          n326 = while {
                            stop <- w929 stop-if-true
                            n327 = call "Get Status.vi"() -> ("function return"=w935:u32, "status out"=w932:i32)  [unwired: 10 in]
                            n328 = Equal?(x=20073 ("status out"), y=w932) -> (x = y?=w931:bool)
                            n329 = Equal?(x=w935, y=20002 ("x")) -> (x = y?=w930:bool)
                            n330 = And(x=w931, y=w930) -> (x .and. y?=w929:bool)
                          }
                        }
                        frame #2 {
                          n331 = local read "Exposure"() -> (w938:sgl)
                          n332 = Divide(x=w938, y=sgl 1000.0) -> (x/y=w937:sgl)
                          n333 = call "Set Exposure Time.vi"("time"=w937) -> ()  [unwired: 10 in, 1 out]
                        }
                        frame #3 {
                          n334 = call "Start Acquisition.vi"() -> ()  [unwired: 11 in, 1 out]
                        }
                      }
                    }
                  }
                  n335 = local read "Live Mode"() -> (w924:bool)
                  n336 = local read "stop"() -> (w922:bool)
                  n337 = Not(x=w924) -> (.not. x?=w926:bool)
                  n338 = Or(x=w926, y=w922) -> (x .or. y?=w923:bool)
                }
              }
              frame #6 {
                n339 = call "Abort Acquisition.vi"() -> ()  [unwired: 11 in, 1 out]
              }
              frame #7 {
                n340 = property on="Exposure" class="DigNum (strict)"("DisabledEnum"=T13."Disabled and Grayed Out" ("Disabled")) -> ()  [unwired: 2 in, 2 out]
              }
            }
          }
        }
        n341 = event shown="[0] Timeout" {
          selector: _ -> [_]
          dyn-events: _ -> [_]
          timeout: 2000 -> [_]
          event Timeout {
            n342 = event-data() -> ()  [unwired: 1 in, 3 out]
            n343 = call "Get Temperature F.vi"() -> ("temperature out"=w827:sgl)  [unwired: 10 in, 1 out]
            n344 = local write "Camera Temperature"(w827) -> ()
          }
        }
        n345 = local read "stop"() -> (w826:bool)
      }
    }
    frame #2 {
      w944 = u32 20002  # DRV Return Success
      n346 = call "Shut Down.vi"() -> ("function return"=w941:u32)  [unwired: 11 in]
      n347 = Equal?(x=w944, y=w941) -> (x = y?=w943:bool)
      n348 = case shown="False" w943 {
        tunnel: [errorcluster {"status"=FALSE, "code"=0, "source"=""} ("error constant") w951] -> w942
        tunnel: w941 -> [_ w949]
        tunnel: w940 -> [_ w950]
        frame True {
        }
        frame False {
          n349 = call "AndorConvertErrCodeToMessage.vi"("function return"=w949, "Array"=w950) -> ("Element Return"=w948:cluster{i32, string})  [unwired: 8 in, 1 out]
          n350 = Unbundle(w948) -> (w947:i32, w946:string)
          n351 = Bundle(cluster=errorcluster {"status"=FALSE, "code"=0, "source"=""} ("error constant"), "status"=TRUE, "code"=w947, "source"=w946) -> (w951:errorcluster)
        }
      }
    }
  }
  n352 = Merge Errors(w4, w5) -> (w1:errorcluster)
  n353 = case shown="No Error" w1 {
    frame No Error {
      n354 = property on="Info" class="Str"("Value"="Disconnection successful" ("Info")) -> ()  [unwired: 2 in, 2 out]
    }
    frame Error {
      n355 = property on="Info" class="Str"("Value"="Disconnection failed.\nPlease restart microscope components and LabVIEW" ("Info")) -> ()  [unwired: 2 in, 2 out]
    }
  }
  n356 = property on="stop" class="Bool (strict)"(error in=w1, "Value"=FALSE ("stop")) -> (error out=→"error out":errorcluster)  [unwired: 1 in, 1 out]
